vi "Main.vi"(11 "Module Admin":refnum<class "Delacor_lib_QMH_Module Admin.lvclass">) -> ()   [LabVIEW 2020, in "Acquisition.lvlib"]
doc: "This template is based off of the Queued Message Handler design pattern and the Queued Message Handler project template that ships with LabVIEW.\n\nThe main difference is that the queue is private to this module and communication between modules is performed via Broadcast and Request events.\n\nRequest events are wrapped in public API methods and are handled in the Event Handling Loop (EHL) of this VI. Any module can register for Broadcast events sent by this module. The EHL generates messages based on user interface actions.\n\nThe Message Handling Loop (MHL) processes messages generated by the EHL, or by other messages. The messages are string values, so new messages can be added easily to the Message Cases case structure in the MHL. Each message cluster can also provide an optional value for Message Data, which is a variant that can be converted to whatever message-specific data is required.\n_____\nBased on DQMH Project Template 4.0.0.47.\n_____\nBased on DQMH Project Template 7.0.1.1316."
uses:
  Acquisition.lvlib
  Module Data--cluster.ctl
  <vilib>/Delacor/Delacor QMH/Libraries/Message Queue_class/Delacor_lib_QMH_Message Queue.lvclass
  <vilib>/Delacor/Delacor QMH/Libraries/Message Queue_class/Delacor_lib_QMH_Enqueue Message (Single).vi
  <vilib>/Delacor/Delacor QMH/Libraries/Module Admin_class/Delacor_lib_QMH_Module Admin.lvclass
  Stop Argument--cluster.ctl
  <vilib>/Utility/miscctls.llb/LVPointTypeDef.ctl
  Stop Acquiring Argument--cluster.ctl
  CML Shared/Signal Type--enum.ctl
  CML Shared/CML Shared.lvlib
  Settings Editor/Settings Editor.lvlib
  Logger/Logger.lvlib
  CML Shared/Calibration Values--cluster.ctl
  Settings Editor/Settings--cluster.ctl
  Settings Editor/Update Application Settings (Reply Payload)--cluster.ctl
  Start Acquiring Argument--cluster.ctl
  Start Acquiring (Reply Payload)--cluster.ctl
  <vilib>/Peloton/Peloton Config/DCFG Framework/Peloton_lib_DCFG Framework.lvlib
  Configuration/Configuration.lvclass
  Configuration/Configuration--cluster.ctl
  <vilib>/Peloton/Peloton Config/DCFG Framework/Configuration_class/Configuration.lvclass
panel:
  out "Settings":T1
  out "Graph Data":waveform(dbl)[](array[waveform])
  out "error out":errorcluster
  # "This is a headless module. Show its panel to confirm that the Settings are updated correctly and other debugging tasks. Use the Settings Editor to change the settings for this module."
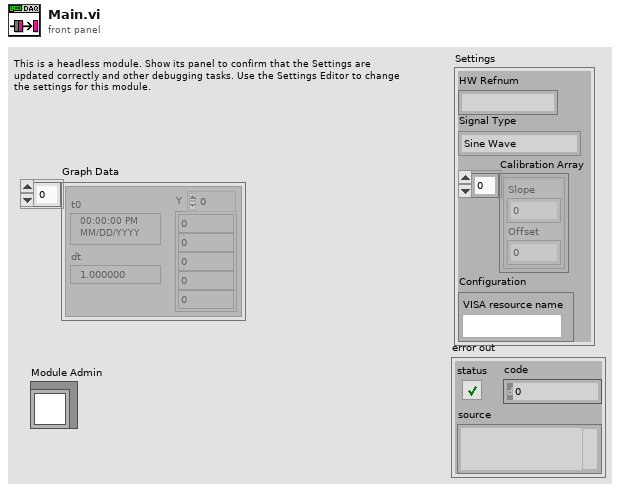
[diagram p1: front panel]
types:
  T1 = typedef "Acquisition.lvlib/Module Data--cluster.ctl" = cluster{"HW Refnum":string, "Signal Type":T2, "Calibration Array":T3[], "Configuration":T4}
  T2 = typedef "CML Shared.lvlib/Signal Type--enum.ctl" = enum16{"Sine Wave", "Square with Noise"}
  T3 = typedef "CML Shared.lvlib/Calibration Values--cluster.ctl" = cluster{"Slope":dbl, "Offset":dbl}
  T4 = typedef "Acquisition.lvlib/Configuration.lvclass/Configuration--cluster.ctl" = cluster{"VISA resource name":refnum<visa-resource-name>}
  T5 = typedef "Settings Editor.lvlib/Broadcast Events--cluster.ctl" = cluster{"Module Did Init":refnum<user-event>, "Status Updated":refnum<user-event>, "Error Reported":refnum<user-event>, "Module Did Stop":refnum<user-event>, "Update Module Execution Status":refnum<user-event>, "Application Settings Updated":refnum<user-event>}
  T6 = typedef "Peloton_lib_DCFG Framework.lvlib/Broadcast Events--cluster.ctl" = cluster{"Module Did Init":refnum<user-event>, "Status Updated":refnum<user-event>, "Error Reported":refnum<user-event>, "Module Did Stop":refnum<user-event>, "Update Module Execution Status":refnum<user-event>, "View Changed":refnum<user-event>, "Main Window Closed":refnum<user-event>, "Configuration Committed":refnum<user-event>, "Configuration Canceled":refnum<user-event>, "Views List Updated":refnum<user-event>, "Config Folder Path Updated":refnum<user-event>}
  T7 = typedef "Acquisition.lvlib/Request Events--cluster.ctl" = cluster{"Stop Module":refnum<user-event>, "Show Panel":refnum<user-event>, "Hide Panel":refnum<user-event>, "Get Module Execution Status":refnum<user-event>, "Show Diagram":refnum<user-event>, "Stop Acquiring":refnum<user-event>, "Wakeup Helper Loop":refnum<user-event>, "Change Settings":refnum<user-event>, "Calibrate DAQ":refnum<user-event>, "Start Acquiring":refnum<user-event>}
  T8 = enum32{"invalid lock state", "Not Locked", "Locked (No Password)", "Password-protected"}
  T9 = typedef "Acquisition.lvlib/Stop Argument--cluster.ctl" = cluster{"Origin":string, "Exit via Stop Module Req?":bool, "Wait for Module to stop?":bool}
  T10 = typedef "Acquisition.lvlib/Start Acquiring Argument--cluster.ctl" = cluster{"Wait Notifier":refnum<notifier>, "wait for reply":bool}
  T11 = typedef "Acquisition.lvlib/Stop Acquiring Argument--cluster.ctl" = cluster{"Boolean":bool}
  T12 = typedef "Settings Editor.lvlib/Update Application Settings (Reply Payload)--cluster.ctl" = cluster{"Settings":T13, "error":errorcluster}
  T13 = typedef "Settings Editor.lvlib/Settings--cluster.ctl" = cluster{"Signal Type":T2, "Calibration Array":T3[], "Log File Base Path":path}
  T14 = typedef "LVPointTypeDef.ctl" = cluster{"Horizontal":i16, "Vertical":i16}
  T15 = enum32{"Invalid", "Standard", "Closed", "Hidden", "Minimized", "Maximized"}
  T16 = typedef "Acquisition.lvlib/Start Acquiring (Reply Payload)--cluster.ctl" = cluster{"HW ID":string, "error":errorcluster}
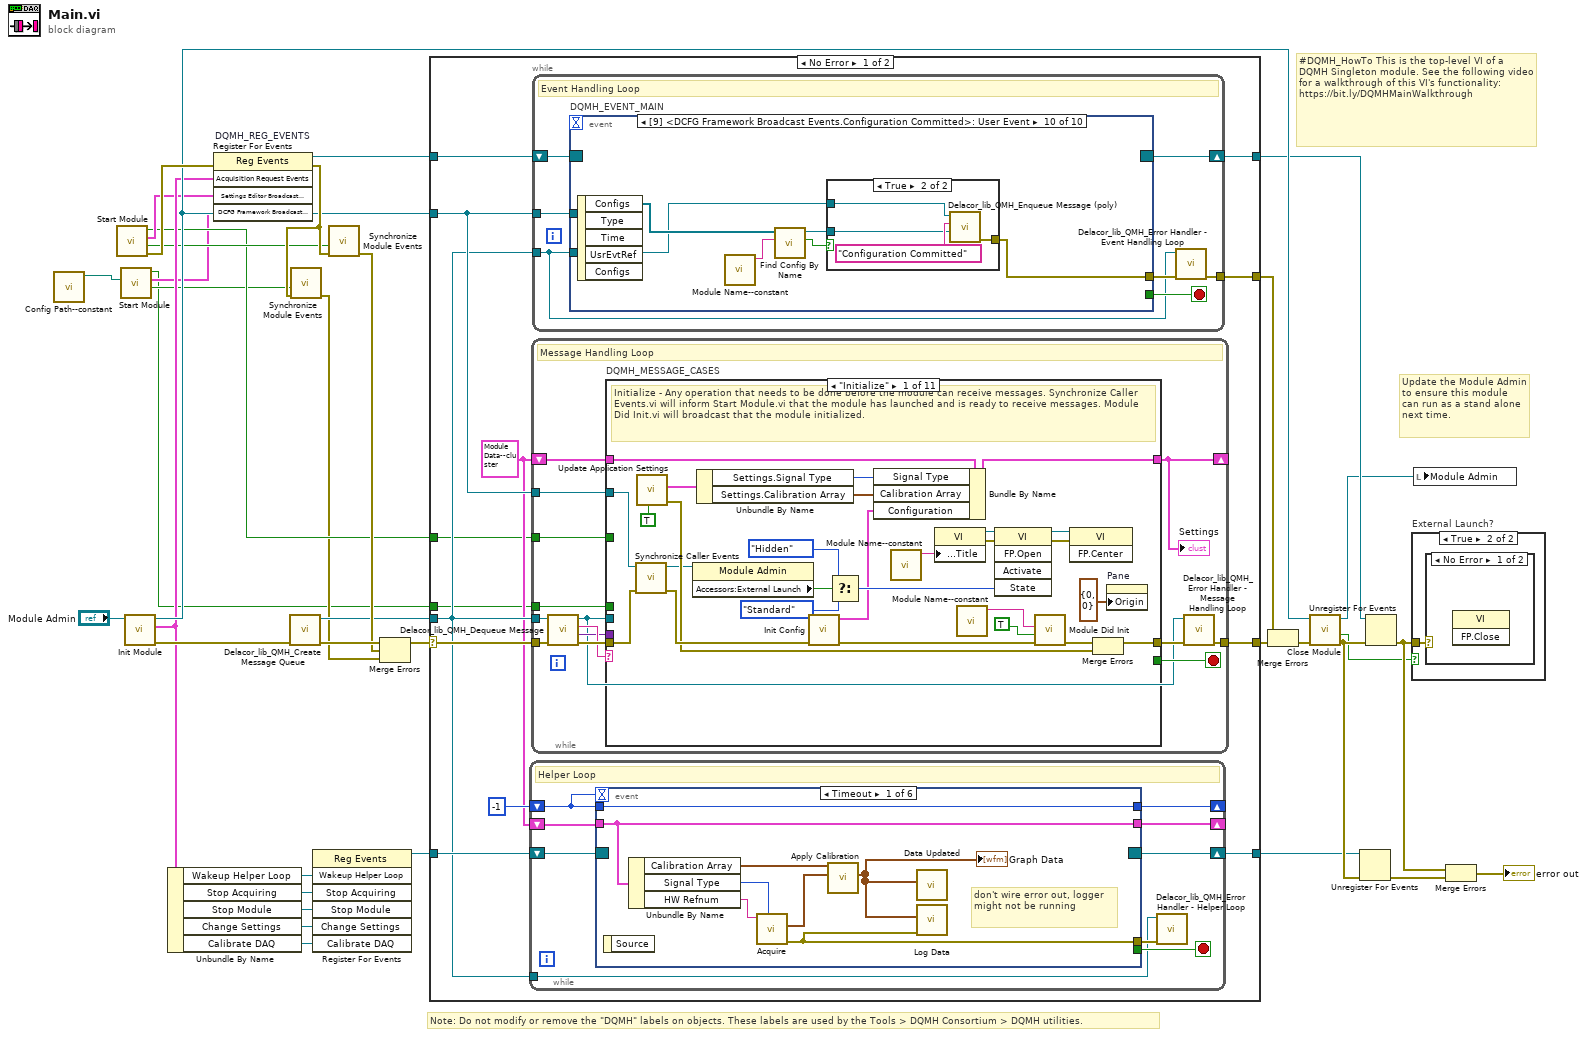
[diagram p0: block diagram]
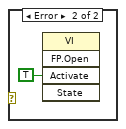
[diagram p3: hidden frame]
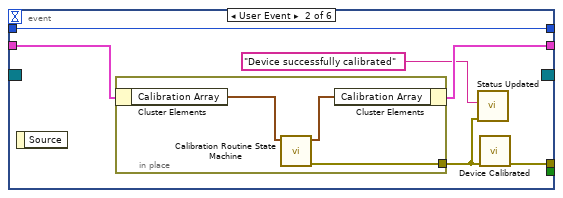
[diagram p4: hidden frame]
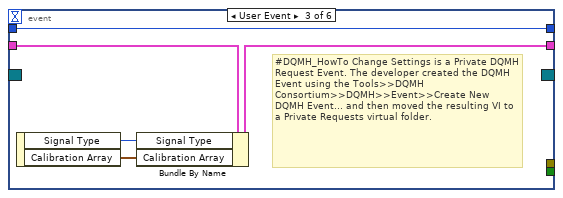
[diagram p5: hidden frame]
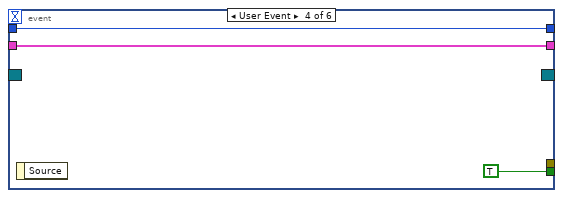
[diagram p6: hidden frame]
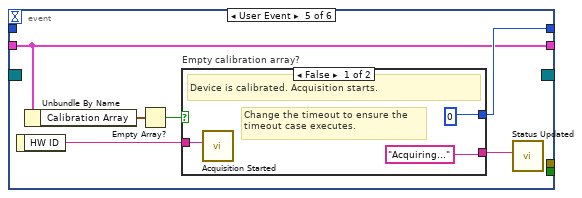
[diagram p7: hidden frame]
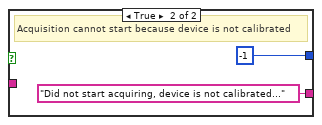
[diagram p8: hidden frame]
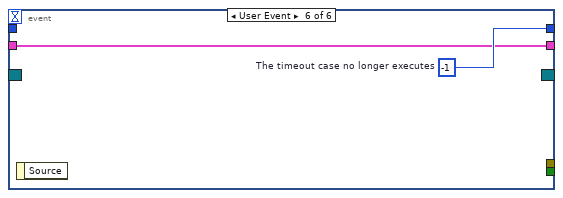
[diagram p9: hidden frame]
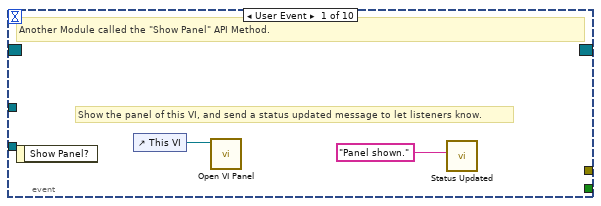
[diagram p10: hidden frame]
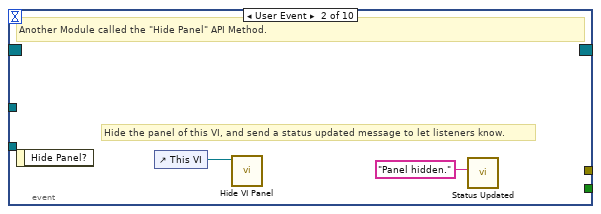
[diagram p11: hidden frame]
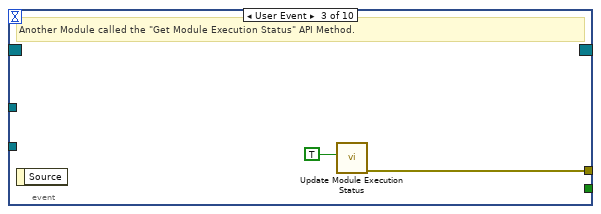
[diagram p12: hidden frame]
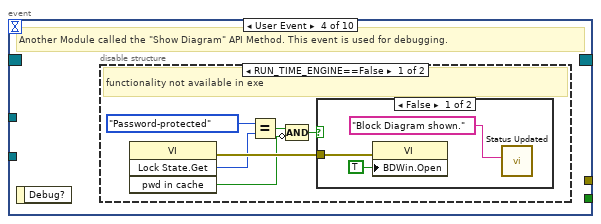
[diagram p13: hidden frame]
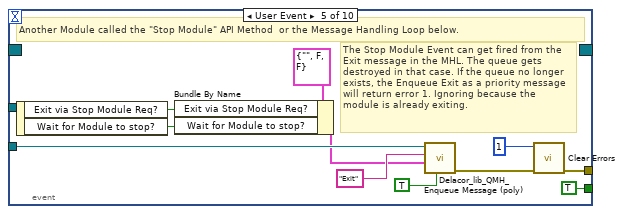
[diagram p16: hidden frame]
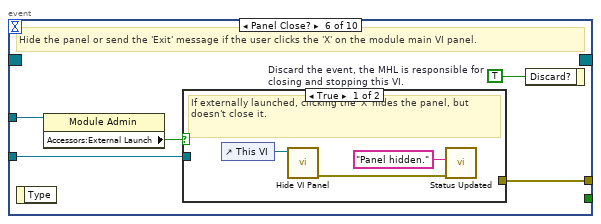
[diagram p17: hidden frame]
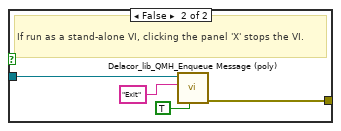
[diagram p18: hidden frame]
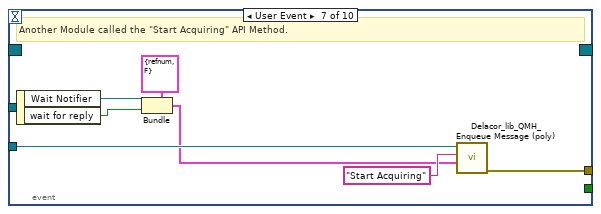
[diagram p19: hidden frame]
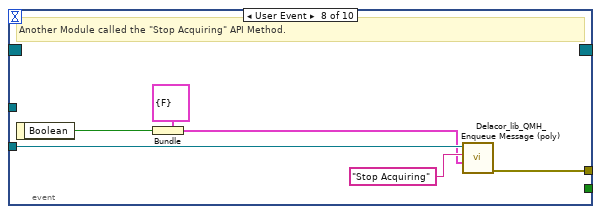
[diagram p20: hidden frame]
diagram:
  # "#DQMH_HowTo This is the top-level VI of a DQMH Singleton module. See the following video for a walkthrough of this VI's functionality: https://bit.ly/DQMHMainWalkthrough"
  # "Note: Do not modify or remove the \"DQMH\" labels on objects. These labels are used by the Tools > DQMH Consortium > DQMH utilities."
  # "Update the Module Admin to ensure this module can run as a stand alone next time."
  n1 = call "Config Path--constant.vi"() -> ("File Path"=w1:path)  [unwired: 11 in]
  n2 = call <vilib>:"Start Module.vi"() -> ("error out"=w29:errorcluster, "Wait for Event Sync?"=w10:bool, "Settings Editor Broadcast Events"=w11:T5, "Module Was Already Running?"=w6:bool)  [unwired: 8 in]
  n3 = call <vilib>:"Start Module.vi"("Config Folder"=w1) -> ("Wait for Event Sync?"=w4:bool, "DCFG Framework Broadcast Events"=w5:T6, "Module Was Already Running?"=w2:bool)  [unwired: 7 in, 1 out]
  n4 = call "Init Module.vi"("Singleton Module Admin in"="Module Admin") -> ("error out"=w35:errorcluster, "Acquisition Request Events"=w16:T7, "Singleton Module Admin out"=w23:refnum<class "Delacor_lib_QMH_Module Admin.lvclass">)  [unwired: 8 in]
  n5 = Unbundle By Name(w16) -> ("Wakeup Helper Loop"=w12:refnum<user-event>, "Stop Acquiring"=w15:refnum<user-event>, "Stop Module"=w14:refnum<user-event>, "Change Settings"=w9:refnum<user-event>, "Calibrate DAQ"=w8:refnum<user-event>)
  n6 = register-events "DQMH_REG_EVENTS"(error in=w29, w16, w11, w5) -> (reference out=w21:refnum<event-registration>, error out=w28:errorcluster)  [unwired: 1 in]
  n7 = call <vilib>:"Delacor_lib_QMH_Create Message Queue.vi"("error in"=w35) -> ("error out"=w31:errorcluster, "Message Queue"=w20:refnum<class "Delacor_lib_QMH_Message Queue.lvclass">)  [unwired: 9 in]
  n8 = call <vilib>:"Synchronize Module Events.vi"("error in (no error)"=w28, "Wait for Event Sync?"=w4) -> ("error out"=w3:errorcluster)  [unwired: 9 in]
  n9 = register-events(w12, w15, w14, w9, w8) -> (reference out=w13:refnum<event-registration>)  [unwired: 2 in, 1 out]
  n10 = call <vilib>:"Synchronize Module Events.vi"("error in"=w28, "Wait for Event Sync?"=w10) -> ("error out"=w27:errorcluster)  [unwired: 9 in]
  n11 = Merge Errors(w31, w27, w3) -> (w30:errorcluster)
  n12 = case shown="No Error" w30 {
    selector: w30 -> [w47 w323]
    tunnel: [w49 w322] -> w36
    tunnel: [w46 w321] -> w22
    tunnel: w21 -> [w45 w321]
    tunnel: w20 -> [w41 w314]
    tunnel: [w48 _] -> w34
    tunnel: w23 -> [w44 w317]
    tunnel: w13 -> [w42 w316]
    tunnel: [w39 w316] -> w7
    tunnel: w6 -> [w38 w315]
    tunnel: w2 -> [w37 w313]
    frame No Error {
      w40 = T1 {"HW Refnum"="", "Signal Type"=enum."Sine Wave", "Calibration Array"=[{"Slope"=1.0, "Offset"=0.0}], "Configuration"={"VISA resource name"=""}} ("Data Cluster")
      n13 = while {
        shift-right: [w57] -> _
        shift-left: -1 -> [w56]
        tunnel: w41 -> [w50]
        shift-right: [w53] -> _
        shift-left: w40 -> [w52]
        shift-right: [w51] -> w39
        shift-left: w42 -> [w55]
        stop <- w54 stop-if-true
        # "Helper Loop"
        n14 = event shown="[0] Timeout" {
          selector: w55 -> [_ _ _ _ _ _]
          dyn-events: [_ _ _ _ _ _] -> w51
          timeout: w56 -> [_ _ _ _ _ _]
          tunnel: [w65 w70 w80 w83 w88 w96] -> w57
          tunnel: w56 -> [w65 w70 w80 w83 _ _]
          tunnel: [_ _ _ TRUE _ _] -> w54
          tunnel: [w66 w72 _ _ _ _] -> w58
          tunnel: [w62 w68 w78 w81 w85 w95] -> w53
          tunnel: w52 -> [w62 w69 w79 w81 w85 w95]
          event Timeout {
            # "don't wire error out, logger might not be running"
            n15 = event-data() -> ()  [unwired: 1 in, 1 out]
            n16 = Unbundle By Name(w62) -> ("Calibration Array"=w60:T3[], "Signal Type"=w64:T2, "HW Refnum"=w63:string)
            n17 = call "Acquire.vi"("Signal Type"=w64, "HW ID in"=w63) -> ("error out"=w66:errorcluster, "Graph Data"=w61:waveform(dbl)[])  [unwired: 7 in, 1 out]
            n18 = call "Apply Calibration.vi"("Graph Data"=w61, "Calibration Array"=w60) -> ("Calibrated Data"=w59:waveform(dbl)[])  [unwired: 9 in]
            "Graph Data" <- w59
            n19 = call "Data Updated.vi"("Graph Data"=w59) -> ()  [unwired: 10 in, 1 out]
            n20 = call "Log Data.vi"("error in"=w66, "Waveforms"=w59) -> ()  [unwired: 9 in, 1 out]
          }
          event User Event {
            n21 = event-data() -> ()  [unwired: 1 in, 1 out]
            n22 = in-place {
              in-place-border: [w75] -> w71
              n23 = in-place-cluster #1(w69) -> ("Calibration Array"=w74:T3[])
              n24 = call "Calibration Routine State Machine.vi"("Calibration Array in"=w74) -> ("error out"=w75:errorcluster, "Calibration Array out"=w73:T3[])  [unwired: 9 in]
              n25 = in-place-cluster #1("Calibration Array"=w73) -> (w68:T1)
            }
            n26 = call "Status Updated.vi"("error in"=w71, "Status"="Device successfully calibrated") -> ()  [unwired: 9 in, 1 out]
            n27 = call "Device Calibrated.vi"("error in"=w71) -> ("error out"=w72:errorcluster)  [unwired: 10 in]
          }
          event User Event {
            # "#DQMH_HowTo Change Settings is a Private DQMH Request Event. The developer created the DQMH Event using the Tools>>DQMH Consortium>>DQMH>>Event>>Create New DQMH Event... and then moved the resulting VI to a Private Requests virtual folder."
            n28 = event-data() -> ("Signal Type"=w77:T2, "Calibration Array"=w76:T3[])  [unwired: 1 in]
            n29 = Bundle By Name(cluster=w79, "Signal Type"=w77, "Calibration Array"=w76) -> (w78:T1)
          }
          event User Event {
            n30 = event-data() -> ()  [unwired: 1 in, 1 out]
          }
          event User Event {
            n31 = event-data() -> ("HW ID"=w86:string)  [unwired: 1 in]
            n32 = Unbundle By Name(w85) -> ("Calibration Array"=w84:T3[])
            n33 = Empty Array?(array=w84) -> (empty?=w89:bool)
            n34 = case "Empty calibration array?" shown="False" w89 {
              tunnel: ["Acquiring..." ("Status") "Did not start acquiring, device is not calibrated..." ("Status")] -> w87
              tunnel: [0 -1] -> w88
              tunnel: w86 -> [w92 _]
              frame False {
                # "Change the timeout to ensure the timeout case executes."
                # "Device is calibrated. Acquisition starts."
                n35 = call "Acquisition Started.vi"("HW ID"=w92) -> ()  [unwired: 10 in, 1 out]
              }
              frame True {
                # "Acquisition cannot start because device is not calibrated"
              }
            }
            n36 = call "Status Updated.vi"("Status"=w87) -> ()  [unwired: 10 in, 1 out]
          }
          event User Event {
            w96 = -1  # The timeout case no longer executes
            n37 = event-data() -> ()  [unwired: 1 in, 1 out]
          }
        }
        n38 = call-dynamic "Delacor_lib_QMH_Error Handler - Helper Loop.vi"("error in"=w58, "Message Queue in"=w50) -> ()  [unwired: 8 in, 2 out]
      }
      n39 = while {
        tunnel: w41 -> [w175]
        shift-right: [w179] -> _
        shift-left: w40 -> [w180]
        tunnel: w47 -> [w183]
        tunnel: [w181] -> w49
        tunnel: w44 -> [w173]
        tunnel: w38 -> [w172]
        tunnel: w37 -> [w171]
        stop <- w178 stop-if-true
        # "Message Handling Loop"
        n40 = call-dynamic "Delacor_lib_QMH_Dequeue Message.vi"("error in"=w183, "Message Queue in"=w175) -> ("error out"=w182:errorcluster, "Message Data"=w176:variant, "Message"=w177:string, "Message Queue out"=w174:refnum<class "Delacor_lib_QMH_Message Queue.lvclass">)  [unwired: 6 in]
        n41 = case "DQMH_MESSAGE_CASES" shown="\"Initialize\"" w177 {
          selector: w177 -> [_ _ _ _ _ _ _ _ _ w300 _]
          tunnel: w174 -> [_ _ _ _ _ _ _ w259 w285 _ _]
          tunnel: w182 -> [w209 w213 w226 w240 w250 w253 w255 w266 w292 w303 w312]
          tunnel: [w206 w213 w224 w238 w248 w252 w255 w262 w286 w304 w309] -> w184
          tunnel: w180 -> [w196 w212 w214 w235 w246 w251 w254 w261 w277 w301 w311]
          tunnel: [w191 w212 w222 w235 w246 w251 w254 w261 w277 w301 w310] -> w179
          tunnel: [_ _ _ _ _ _ _ _ w284 _ _] -> w178
          tunnel: w176 -> [_ _ w221 w237 w247 _ _ w260 w283 _ w308]
          tunnel: w173 -> [w197 _ _ _ _ _ _ w258 w278 _ _]
          tunnel: w172 -> [_ _ _ _ _ _ _ _ w275 _ _]
          tunnel: w171 -> [_ _ _ _ _ _ _ _ w273 _ _]
          frame "Initialize" {
            # "Initialize - Any operation that needs to be done before the module can receive messages. Synchronize Caller Events.vi will inform Start Module.vi that the module has launched and is ready to receive messages. Module Did Init.vi will broadcast that the module initialized."
            n42 = call "Synchronize Caller Events.vi"("error in"=w209, "Singleton Module Admin in"=w197) -> ("error out"=w208:errorcluster, "Singleton Module Admin out"=w193:refnum<class "Delacor_lib_QMH_Module Admin.lvclass">)  [unwired: 8 in]
            n43 = call "Update Application Settings.vi"("wait for reply (T)"=TRUE) -> ("error out"=w205:errorcluster, "Reply Payload"=w190:T12)  [unwired: 8 in, 1 out]
            n44 = property on="Property Node" class="Module Admin"(reference=w193) -> ("Accessors:External Launch"=w201:bool)  [unwired: 1 in, 2 out]
            n45 = Unbundle By Name(w190) -> ("Settings.Signal Type"=w189:T2, "Settings.Calibration Array"=w188:T3[])
            n46 = call "Init Config.vi"("error in"=w208) -> ("error out"=w186:errorcluster, "Configuration"=w185:T4)  [unwired: 9 in]
            n47 = Select(t=T15."Hidden" ("State"), s=w201, f=T15."Standard" ("State")) -> (s? t:f=w198:T15)
            n48 = Bundle By Name(cluster=w196, "Signal Type"=w189, "Calibration Array"=w188, "Configuration"=w185) -> (w191:T1)
            n49 = call "Module Name--constant.vi"() -> ("Module Name"=w204:string)  [unwired: 11 in]
            n50 = property on="Property Node" class="VI"("Front Panel.Title"=w204) -> (reference out=w203:refnum<vi>, error out=w211:errorcluster)  [unwired: 2 in]
            n51 = call "Module Name--constant.vi"() -> ("Module Name"=w194:string)  [unwired: 11 in]
            n52 = invoke on="Invoke Node" class="VI" method="FP.Open"(reference=w203, error in=w211, "State"=w198) -> (reference out=w202:refnum<vi>, error out=w210:errorcluster)  [unwired: 2 in, 3 out]
            n53 = call "Module Did Init.vi"("error in"=w186, "Initialized?"=TRUE, "Origin"=w194) -> ("error out"=w207:errorcluster)  [unwired: 8 in]
            n54 = invoke on="Invoke Node" class="VI" method="FP.Center"(reference=w202, error in=w210) -> ()  [unwired: 1 in, 3 out]
            n55 = Merge Errors(w207, w205) -> (w206:errorcluster)
            n56 = property on="Pane" class="Pane"("Origin"=T14 {"Horizontal"=0, "Vertical"=0}) -> ()  [unwired: 2 in, 2 out]
          }
          frame "---Module Specific---" {
            # "Separator -- The following cases handle messages specific to this Module."
          }
          frame "Start Acquiring" {
            # "Requests Acquisition Module to start acquiring."
            n57 = Variant To Data(error in=w226, type=T10 {"Wait Notifier"=refnum, "wait for reply"=FALSE} ("Start Acquisition Argument"), Variant=w221) -> (data=w219:T10, error out=w223:errorcluster)
            n58 = in-place {
              in-place-border: [w232] -> w225
              in-place-border: w223 -> [w231]
              in-place-border: [w227] -> w215
              n59 = in-place-cluster #2(w214) -> ("HW Refnum"=w228:string)
              n60 = call "Initialize Hardware References.vi"("error in"=w231, "HW Refnum in"=w228) -> ("error out"=w230:errorcluster, "HW Refnum out"=w229:string)  [unwired: 8 in]
              n61 = call "Configure Hardware.vi"("error in"=w230, "HW Refnum in"=w229) -> ("error out"=w232:errorcluster, "HW Refnum out"=w227:string)  [unwired: 8 in]
              n62 = in-place-cluster #2("HW Refnum"=w227) -> (w222:T1)
            }
            n63 = Unbundle By Name(w219) -> ("Wait Notifier"=w218:refnum<notifier>)
            n64 = call "Wakeup Helper Loop.vi"("error in"=w225, "HW ID"=w215) -> ("error out"=w224:errorcluster)  [unwired: 9 in]
            n65 = Bundle By Name(cluster=T16 {"HW ID"="", "error"={"status"=FALSE, "code"=0, "source"=""}} ("Start Acquisition (Reply Payload)"), "HW ID"=w215, "error"=w225) -> (w217:T16)
            n66 = Send Notification(notification=w217, notifier=w218) -> ()  [unwired: 1 in, 2 out]
          }
          frame "Stop Acquiring" {
            # "Requests the Acquisition Module to stop acquiring"
            n67 = Variant To Data(error in=w240, type=T11 {"Boolean"=FALSE} ("Stop Acquiring Argument"), Variant=w237) -> (error out=w239:errorcluster)  [unwired: 1 out]
            n68 = Unbundle By Name(w235) -> ("HW Refnum"=w234:string)
            n69 = call "Stop Acquisition.vi"("error in"=w239, "HW Refnum"=w234) -> ("error out"=w238:errorcluster)  [unwired: 9 in]
            n70 = call "Acquisition Stopped.vi"("error in"=w238) -> ()  [unwired: 10 in, 1 out]
            n71 = call "Status Updated.vi"("error in"=w238, "Status"="Acquisition Stopped") -> ()  [unwired: 9 in, 1 out]
          }
          frame "Update Settings" {
            # "Send the Change Settings event to the helper loop."
            # "The Settings Editor broadcasted that the settings have changed."
            n72 = Variant To Data(error in=w250, type=T12 {"Settings"={"Signal Type"=enum."Sine Wave", "Calibration Array"=[], "Log File Base Path"=path ""}, "error"={"status"=FALSE, "code"=0, "source"=""}} ("Settings Updated Argument"), Variant=w247) -> (data=w244:T12, error out=w249:errorcluster)
            n73 = Unbundle By Name(w244) -> ("Settings.Signal Type"=w243:T2, "Settings.Calibration Array"=w241:T3[])
            n74 = call "Change Settings.vi"("error in"=w249, "Calibration Array"=w241, "Signal Type"=w243) -> ("error out"=w248:errorcluster)  [unwired: 8 in]
            n75 = call "Status Updated.vi"("error in"=w248, "Status"="Settings Updated") -> ()  [unwired: 9 in, 1 out]
          }
          frame "---Copy This Frame---" {
            # "Duplicate this frame when creating new messages.  Change this comment in the duplicated frame to describe this message."
            n76 = Merge Errors(w253) -> (w252:errorcluster)
          }
          frame "---Exit and Error Handling---" {
            # "Separator - The following cases handle errors and exit messages."
          }
          frame "Error" {
            # "Error - Check the error message data and respond accordingly. This message is sent by the \"Error Handler\" VIs at the end of each loop in this application."
            n77 = property on="Property Node" class="Module Admin"(reference=w258) -> ("Accessors:External Launch"=w257:bool)  [unwired: 1 in, 2 out]
            n78 = Variant To Data(error in=w266, type=errorcluster {"status"=FALSE, "code"=0, "source"=""} ("error constant"), Variant=w260) -> (data=w256:errorcluster, error out=w264:errorcluster)
            n79 = local write "error out"(w256) -> ()
            n80 = call "Error Reported.vi"("Error"=w256) -> ()  [unwired: 10 in, 1 out]
            n81 = case shown="False" w257 {
              tunnel: [w271 _] -> w263
              tunnel: w259 -> [w269 _]
              tunnel: w256 -> [w270 _]
              frame False {
                n82 = disable-structure shown="Default" {
                  disable-tunnel: w270 -> [w272 _]
                  frame condition #0 (active) {
                    # "If the module is running standalone, then pop up an error dialog and call the \"Exit\" message."
                    n83 = call <vilib>:"Simple Error Handler.vi"("error in (no error)"=w272) -> ()  [unwired: 4 in, 5 out]
                  }
                  frame condition #1 {
                    # "To prevent the Simple Error Handler VI from being loaded (e.g. when deploying to a Real-Time target), add the Conditional Disable Symbol \"DQMH_Disable_SEH\" to your project and set it to TRUE."
                  }
                }
                n84 = call-poly <vilib>:"Delacor_lib_QMH_Enqueue Message (poly).vi"("Priority Message? (F)"=TRUE, "Message"="Exit", "Message Queue in"=w269) -> ("error out"=w271:errorcluster)  [unwired: 7 in, 1 out]
              }
              frame True {
                # "If the module was launched externally, calling the Error Reported broadcast VI is the only action performed by the \"Error\" message. The module's caller can then process the error appropriately."
              }
            }
            n85 = Merge Errors(w264, w263) -> (w262:errorcluster)
          }
          frame "Exit" {
            w284 = TRUE  # Stop the VI
            # "Release the message queue reference"
            # "Exit - Exit the application."
            n86 = Variant To Data(error in=w292, type=T9 {"Origin"="", "Exit via Stop Module Req?"=FALSE, "Wait for Module to stop?"=FALSE} ("Stop Argument"), Variant=w283) -> (data=w280:T9, error out=w289:errorcluster)
            n87 = call <vilib>:"Clear Errors.vi"("error in (no error)"=w289, "specific error code to clear (0: all)"=91 ("91: not all Exit messages will have an argument")) -> ("error out"=w291:errorcluster)  [unwired: 4 in, 1 out]
            n88 = Unbundle By Name(w277) -> ("HW Refnum"=w276:string)
            n89 = control-ref of="This VI"() -> (w279:refnum<vi>)
            n90 = call "Destroy Config.vi"() -> ("error out"=w274:errorcluster)  [unwired: 11 in]
            n91 = case "DCFG_Stop_Case" shown="False" w273 {
              tunnel: w274 -> [_ _]
              frame False {
                n92 = call <vilib>:"Stop Module.vi"() -> ()  [unwired: 11 in, 1 out]
              }
              frame True {
                # "Let DCFG Running if it was already running"
              }
            }
            n93 = call "Handle Exit.vi"("Stop Argument"=w280, "Admin in"=w278, "VI reference"=w279) -> ("error out"=w288:errorcluster)  [unwired: 7 in, 1 out]
            n94 = call "Close Hardware References.vi"("HW Refnum in"=w276) -> ("error out"=w287:errorcluster)  [unwired: 9 in, 1 out]
            n95 = call-dynamic "Delacor_lib_QMH_Release Message Queue.vi"("error in"=w291, "Message Queue"=w285) -> ("error out"=w290:errorcluster)  [unwired: 9 in]
            n96 = case "Settings Editor was\nalready running?" shown="False" w275 {
              frame False {
                n97 = call "Module Name--constant.vi"() -> ("Module Name"=w294:string)  [unwired: 11 in]
                n98 = call <vilib>:"Stop Module.vi"("Wait for Module to Stop? (F)"=TRUE, "Origin"=w294) -> ()  [unwired: 9 in, 1 out]
              }
              frame True {
                # "Another Module stops the Settings Editor"
              }
            }
            n99 = Merge Errors(w290, w288, w287) -> (w286:errorcluster)
            n100 = call "Error Reported.vi"("Error"=w286) -> ()  [unwired: 10 in, 1 out]
          }
          frame Default {
            # "'Default' case only runs if there is a message that isn't defined in any of the other cases.  Output a programming error."
            n101 = call "Module Name--constant.vi"() -> ("Module Name"=w299:string)  [unwired: 11 in]
            n102 = Format Into String(format string="The invalid message string \"%s\" was received in the Message Handling Loop for module \"%s\".", w300, w299) -> (resulting string=w297:string)  [unwired: 2 in, 1 out]
            n103 = call <vilib>:"Error Cluster From Error Code.vi"("show call chain? (False)"=TRUE, "error message (\"\")"=w297, "error code (0)"=1) -> ("error out"=w302:errorcluster)  [unwired: 6 in]
            n104 = Merge Errors(w303, w302) -> (w304:errorcluster)
          }
          frame "Configuration Committed" {
            w306 = refnum<class "Configuration.lvclass"> refnum  # Module_Config_Class
            n105 = Variant To Data(error in=w312, type=w306, Variant=w308) -> (data=w305:refnum<class "Configuration.lvclass">, error out=w309:errorcluster)
            n106 = property on="Property Node" class="Config"(reference=w305) -> ("Accessors:Configuration"=w307:T4)  [unwired: 1 in, 2 out]
            n107 = Bundle By Name(cluster=w311, "Configuration"=w307) -> (w310:T1)
          }
        }
        "Settings" <- w179
        n108 = call-dynamic "Delacor_lib_QMH_Error Handler - Message Handling Loop.vi"("error in"=w184, "Message Queue in"=w174) -> ("dup error in"=w181:errorcluster)  [unwired: 8 in, 1 out]
      }
      n109 = while {
        tunnel: w41 -> [w97]
        shift-right: [w100] -> w46
        shift-left: w45 -> [w101]
        tunnel: [w102] -> w48
        tunnel: w44 -> [w98]
        stop <- w99 stop-if-true
        # "Event Handling Loop"
        n110 = event "DQMH_EVENT_MAIN" shown="[9] <DCFG Framework Broadcast Events.Configuration Committed>: User Event" {
          selector: w101 -> [_ _ _ _ _ _ _ _ _ _]
          dyn-events: [_ _ _ _ _ _ _ _ _ _] -> w100
          timeout: _ -> [_ _ _ _ _ _ _ _ _ _]
          tunnel: [_ _ _ _ TRUE ("Discard?") _ _ _ _ _] -> w99
          tunnel: w97 -> [_ _ _ _ w125 w132 w147 w153 w158 w164]
          tunnel: [_ _ w109 _ w128 w134 w148 w154 w160 w166] -> w103
          tunnel: w98 -> [_ _ _ _ _ w131 _ _ _ _]
          event User Event {
            # "Show the panel of this VI, and send a status updated message to let listeners know."
            # "Another Module called the \"Show Panel\" API Method."
            n111 = event-data() -> ()  [unwired: 1 in, 1 out]
            n112 = control-ref of="This VI"() -> (w105:refnum<vi>)
            n113 = call "Open VI Panel.vi"("VI"=w105) -> ()  [unwired: 10 in, 1 out]
            n114 = call "Status Updated.vi"("Status"="Panel shown." ("format string")) -> ()  [unwired: 10 in, 1 out]
          }
          event User Event {
            # "Hide the panel of this VI, and send a status updated message to let listeners know."
            # "Another Module called the \"Hide Panel\" API Method."
            n115 = event-data() -> ()  [unwired: 1 in, 1 out]
            n116 = control-ref of="This VI"() -> (w107:refnum<vi>)
            n117 = call "Hide VI Panel.vi"("VI"=w107) -> ()  [unwired: 10 in, 1 out]
            n118 = call "Status Updated.vi"("Status"="Panel hidden." ("format string")) -> ()  [unwired: 10 in, 1 out]
          }
          event User Event {
            # "Another Module called the \"Get Module Execution Status\" API Method."
            n119 = event-data() -> ()  [unwired: 1 in, 1 out]
            n120 = call "Update Module Execution Status.vi"("Running?"=TRUE) -> ("error out"=w109:errorcluster)  [unwired: 10 in]
          }
          event User Event {
            # "Another Module called the \"Show Diagram\" API Method. This event is used for debugging."
            n121 = event-data() -> ()  [unwired: 1 in, 1 out]
            n122 = disable-structure shown="RUN_TIME_ENGINE==False" {
              frame condition #0 (active) {
                # "functionality not available in exe"
                n123 = invoke on="Invoke Node" class="VI" method="Lock State.Get"() -> (error out=w115:errorcluster, "Get Lock State"=w114:T8, "pwd in cache"=w111:bool)  [unwired: 4 in, 1 out]
                n124 = Equal?(x=T8."Password-protected", y=w114) -> (x = y?=w112:bool)
                n125 = Compound Arithmetic op=AND(w112, invert w111) -> (w110:bool)
                n126 = case shown="False" w110 {
                  tunnel: w115 -> [w118 _]
                  frame False {
                    n127 = property on="Property Node" class="VI"(error in=w118, "BDWin.Open"=TRUE ("Block Diagram Window:Open")) -> ()  [unwired: 1 in, 2 out]
                    n128 = call "Status Updated.vi"("Status"="Block Diagram shown." ("format string")) -> ()  [unwired: 10 in, 1 out]
                  }
                  frame True {
                    # "Password-protected VI, and the password is not in the cache. Do not show the diagram."
                  }
                }
              }
              frame condition #1 {
              }
            }
          }
          event User Event {
            # "The Stop Module Event can get fired from the Exit message in the MHL. The queue gets destroyed in that case. If the queue no longer exists, the Enqueue Exit as a priority message will return error 1. Ignoring because the module is already exiting."
            # "Another Module called the \"Stop Module\" API Method  or the Message Handling Loop below."
            n129 = event-data() -> ("Exit via Stop Module Req?"=w121:bool, "Wait for Module to stop?"=w120:bool)  [unwired: 1 in]
            n130 = Bundle By Name(cluster=T9 {"Origin"="", "Exit via Stop Module Req?"=FALSE, "Wait for Module to stop?"=FALSE} ("Stop Argument"), "Exit via Stop Module Req?"=w121, "Wait for Module to stop?"=w120) -> (w119:T9)
            n131 = call-poly <vilib>:"Delacor_lib_QMH_Enqueue Message (poly).vi"("Priority Message? (F)"=TRUE, "Message Data"=w119, "Message"="Exit", "Message Queue in"=w125) -> ("error out"=w129:errorcluster)  [unwired: 6 in, 1 out]
            n132 = call <vilib>:"Clear Errors.vi"("error in (no error)"=w129, "specific error code to clear (0: all)"=1) -> ("error out"=w128:errorcluster)  [unwired: 4 in, 1 out]
          }
          event Panel Close? {
            w133 = TRUE  # Discard the event, the MHL is responsible for closing and stopping this VI.
            # "Hide the panel or send the 'Exit' message if the user clicks the 'X' on the module main VI panel."
            n133 = event-data() -> ()  [unwired: 1 in, 1 out]
            n134 = property on="Property Node" class="Module Admin"(reference=w131) -> ("Accessors:External Launch"=w130:bool)  [unwired: 1 in, 2 out]
            n135 = case shown="True" w130 {
              tunnel: w132 -> [_ w140]
              tunnel: [_ w141] -> w134
              frame True {
                # "If externally launched, clicking the 'X' hides the panel, but doesn't close it."
                n136 = control-ref of="This VI"() -> (w137:refnum<vi>)
                n137 = call "Hide VI Panel.vi"("VI"=w137) -> ("error out"=w135:errorcluster)  [unwired: 10 in]
                n138 = call "Status Updated.vi"("error in"=w135, "Status"="Panel hidden." ("format string")) -> ()  [unwired: 9 in, 1 out]
              }
              frame False {
                # "If run as a stand-alone VI, clicking the panel 'X' stops the VI."
                n139 = call-poly <vilib>:"Delacor_lib_QMH_Enqueue Message (poly).vi"("Priority Message? (F)"=TRUE, "Message"="Exit", "Message Queue in"=w140) -> ("error out"=w141:errorcluster)  [unwired: 7 in, 1 out]
              }
            }
            n140 = event-data ("Event Filter Node")("Discard?"=w133) -> ()  [unwired: 1 in, 1 out]
          }
          event User Event {
            # "Another Module called the \"Start Acquiring\" API Method."
            n141 = event-data() -> ("Wait Notifier"=w143:refnum<notifier>, "wait for reply"=w142:bool)  [unwired: 1 in]
            n142 = Bundle(cluster=T10 {"Wait Notifier"=refnum, "wait for reply"=FALSE} ("Start Acquisition Argument"), "Wait Notifier"=w143, "wait for reply"=w142) -> (w144:T10)
            n143 = call-poly <vilib>:"Delacor_lib_QMH_Enqueue Message (poly).vi"("Message Data"=w144, "Message"="Start Acquiring", "Message Queue in"=w147) -> ("error out"=w148:errorcluster)  [unwired: 7 in, 1 out]
          }
          event User Event {
            # "Another Module called the \"Stop Acquiring\" API Method."
            n144 = event-data() -> ("Boolean"=w149:bool)  [unwired: 1 in]
            n145 = Bundle(cluster=T11 {"Boolean"=FALSE} ("Stop Acquiring Argument"), "Boolean"=w149) -> (w150:T11)
            n146 = call-poly <vilib>:"Delacor_lib_QMH_Enqueue Message (poly).vi"("Message Data"=w150, "Message"="Stop Acquiring", "Message Queue in"=w153) -> ("error out"=w154:errorcluster)  [unwired: 7 in, 1 out]
          }
          event User Event {
            n147 = event-data() -> ("Settings"=w155:T13)  [unwired: 1 in]
            n148 = Bundle By Name(cluster=T12 {"Settings"={"Signal Type"=enum."Sine Wave", "Calibration Array"=[], "Log File Base Path"=path ""}, "error"={"status"=FALSE, "code"=0, "source"=""}} ("Settings Updated Argument"), "Settings"=w155) -> (w157:T12)
            n149 = call-poly <vilib>:"Delacor_lib_QMH_Enqueue Message (poly).vi"("Message Data"=w157, "Message"="Update Settings", "Message Queue in"=w158) -> ("error out"=w160:errorcluster)  [unwired: 7 in, 1 out]
          }
          event User Event {
            n150 = event-data() -> ("Configs"=w165:refnum<class "Configuration.lvclass">[])  [unwired: 1 in, 4 out]
            n151 = call "Module Name--constant.vi"() -> ("Module Name"=w163:string)  [unwired: 11 in]
            n152 = call <vilib>:"Find Config By Name.vi"("Config Name"=w163, "All Config Classes"=w165) -> ("Found"=w162:bool, "Configuration"=w161:refnum<class "Configuration.lvclass">)  [unwired: 6 in, 2 out]
            n153 = case shown="True" w162 {
              tunnel: w164 -> [_ w169]
              tunnel: [_ w170] -> w166
              tunnel: w161 -> [_ w167]
              frame False {
              }
              frame True {
                n154 = call-poly <vilib>:"Delacor_lib_QMH_Enqueue Message (poly).vi"("Message Data"=w167, "Message"="Configuration Committed", "Message Queue in"=w169) -> ("error out"=w170:errorcluster)  [unwired: 7 in, 1 out]
              }
            }
          }
        }
        n155 = call-dynamic "Delacor_lib_QMH_Error Handler - Event Handling Loop.vi"("error in"=w103, "Message Queue in"=w97) -> ("dup error in"=w102:errorcluster)  [unwired: 8 in, 1 out]
      }
    }
    frame Error {
      # "Synchronize Caller Events.vi will inform Start Module.vi that the module has launched and will let the code calling Start Module.vi register for broadcasts and would permit the caller receive the broadcast that an error occurred at launch time."
      n156 = call "Synchronize Caller Events.vi"("Singleton Module Admin in"=w317) -> ("error out"=w324:errorcluster)  [unwired: 9 in, 1 out]
      n157 = call-dynamic "Delacor_lib_QMH_Release Message Queue.vi"("error in"=w323, "Message Queue"=w314) -> ("error out"=w322:errorcluster)  [unwired: 9 in]
      n158 = call "Module Name--constant.vi"() -> ("Module Name"=w320:string)  [unwired: 11 in]
      n159 = case "Settings Editor was\nalready running?" shown="False" w315 {
        frame False {
          n160 = call "Module Name--constant.vi"() -> ("Module Name"=w327:string)  [unwired: 11 in]
          n161 = call <vilib>:"Stop Module.vi"("Wait for Module to Stop? (F)"=TRUE, "Origin"=w327) -> ()  [unwired: 9 in, 1 out]
        }
        frame True {
          # "Another Module is\nin charge of stopping Settings Editor"
        }
      }
      n162 = Format Into String(format string="An error occurred during initialization. %s is no longer running.", w320) -> (resulting string=w318:string)  [unwired: 2 in, 1 out]
      n163 = Merge Errors(w322, w324) -> (w325:errorcluster)
      n164 = case "DCFG_Stop_Case" shown="False" w313 {
        frame False {
          n165 = call <vilib>:"Stop Module.vi"() -> ()  [unwired: 11 in, 1 out]
        }
        frame True {
          # "Let DCFG Running if it was already running"
        }
      }
      n166 = call "Error Reported.vi"("Additional Information"=w318, "Error"=w325) -> ()  [unwired: 9 in, 1 out]
    }
  }
  n167 = Merge Errors(w34, w36) -> (w33:errorcluster)
  n168 = call "Close Module.vi"("error in"=w33, "Module Admin in"=w23) -> ("error out"=w26:errorcluster, "External Launch"=w17:bool, "Module Admin out"=w18:refnum<class "Delacor_lib_QMH_Module Admin.lvclass">)  [unwired: 7 in]
  n169 = Unregister For Events(event registration refnum=w7, error in=w26) -> (error out=w24:errorcluster)
  n170 = Unregister For Events(event registration refnum=w22, error in=w26) -> (error out=w32:errorcluster)
  n171 = case "External Launch?" shown="True" w17 {
    tunnel: w32 -> [_ w328]
    frame False {
    }
    frame True {
      n172 = case shown="No Error" w328 {
        frame No Error {
          n173 = invoke on="Invoke Node" class="VI" method="FP.Close"() -> ()  [unwired: 3 in, 3 out]
        }
        frame Error {
          n174 = invoke on="Invoke Node" class="VI" method="FP.Open"("Activate"=TRUE ("Activate?")) -> ()  [unwired: 4 in, 5 out]
        }
      }
    }
  }
  n175 = local write "Module Admin"(w18) -> ()
  n176 = Merge Errors(w32, w24) -> (→"error out":errorcluster)
